vi "Secure-Release Region.vi"(6 "Numeric":dbl, 7 "Action":enum16{"Secure", "Release"}(ring), 8 "error in (no error)":errorcluster, 10 "Control In":T1={"I-O.lvclass"=refnum, "Gantry"=refnum, "Dispenser"="COM1"}, 11 "Workspace in":refnum<class "Component Tray.lvclass">) -> (0 "error out":errorcluster, 1 "Position":i32, 2 "Control Out":T1={"I-O.lvclass"=refnum, "Gantry"=refnum, "Dispenser"="COM1"}, 3 "Workspace out":refnum<class "Component Tray.lvclass">)   [LabVIEW 2021, in "Component Tray.lvclass"]
uses:
  Component Tray.lvclass
  C:/Users/HEP/Documents/GitHub/Gantry/UCSB-Gantry-HEP-main/Classes/Workspace/Fixture.lvclass
  Controller/Controllers.ctl
  Controller/I-O/I-O.lvclass
  C:/Program Files (x86)/Aerotech/A3200/LabVIEW/2010/Bin/Aerotech.A3200.dll
  Program Files (x86)/Aerotech/A3200/LabVIEW/2010/Bin/Aerotech.A3200.dll
  Fixture.lvclass/Fixture.ctl
  Read Gantry Region.vi
  Read Position.vi
  Fixture.lvclass
  Controller/Motion/Motion.lvclass
  Controller/Controller.lvclass
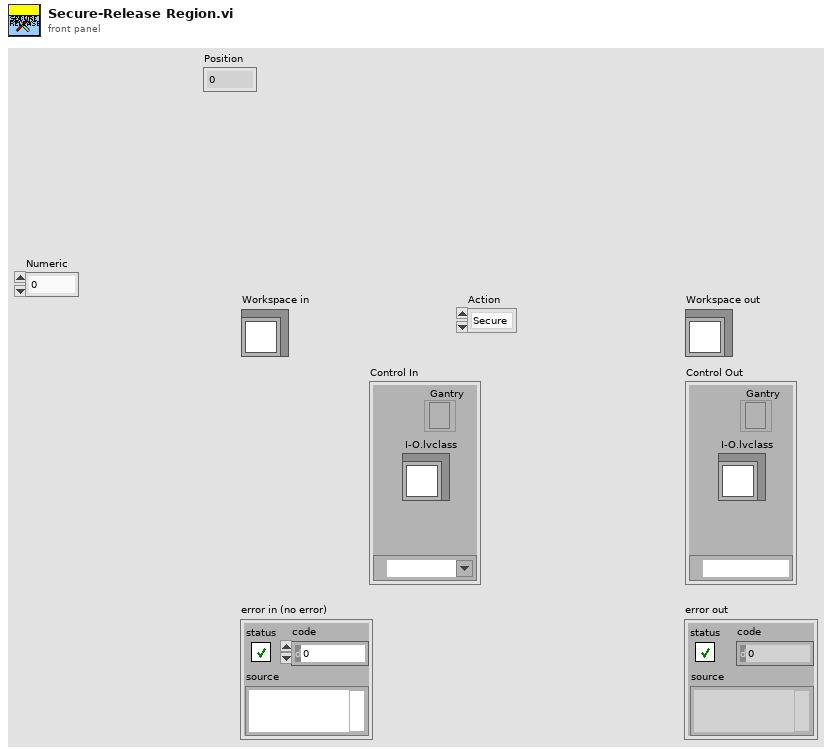
[diagram p1: front panel]
types:
  T1 = typedef "Controller.lvclass/Controllers.ctl" = cluster{"I-O.lvclass":refnum<class "I-O.lvclass">, "Gantry":refnum<k24>, "Dispenser":refnum<visa-resource-name>}
  T2 = typedef "I-O.lvclass/Pin Map.ctl" = cluster{"Region Valves":i32[], "Extra Valves":dbl[][][], "Tool Primary Valve":i32, "Tool Secondary Valve":i32, "Region Sensors":i32[], "Extra Sensors":dbl[][][], "Tool Primary Sensor":dbl, "Tool Secondary Sensor":dbl, "Compression Sensor":dbl, "5V":i32, "Dispenser Sensor":dbl}
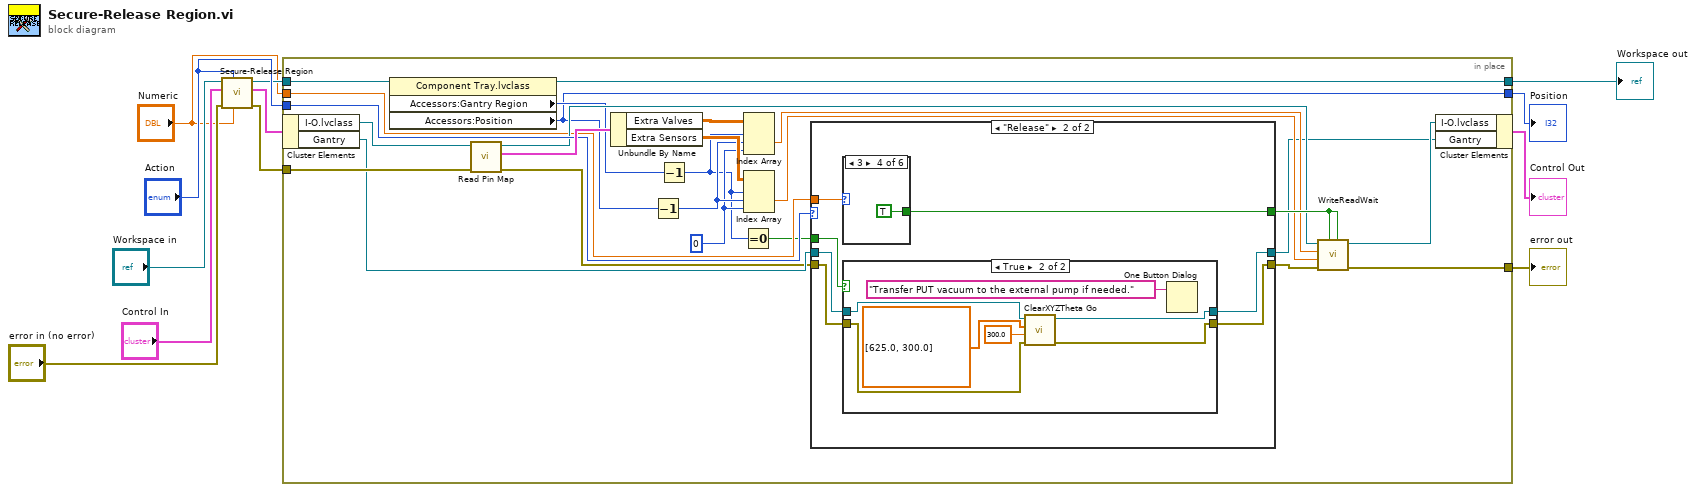
[diagram p0: block diagram]
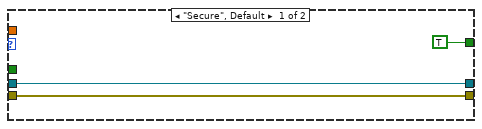
[diagram p2: hidden frame]
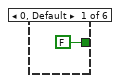
[diagram p4: hidden frame]
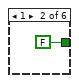
[diagram p5: hidden frame]
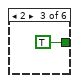
[diagram p6: hidden frame]
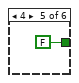
[diagram p7: hidden frame]
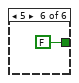
[diagram p8: hidden frame]
diagram:
  n1 = call-parent "Secure-Release Region.vi"("Test Run Number"="Numeric", "Action"="Action", "error in (no error)"="error in (no error)", "Control In"="Control In", "Fixture in"="Workspace in") -> ("error out"=w2:errorcluster, "Control Out"=w9:T1, "Fixture out"=w6:refnum<class "Component Tray.lvclass">)  [unwired: 3 in, 1 out]
  n2 = in-place {
    in-place-border: "Action" -> [w34]
    in-place-border: w6 -> [w31]
    in-place-border: [w26] -> w5
    in-place-border: [w22] -> w4
    in-place-border: "Numeric" -> [w21]
    in-place-border: w2 -> [w19]
    in-place-border: [w18] -> w1
    w23 = 0
    n3 = in-place-cluster #1(w9) -> ("I-O.lvclass"=w36:refnum<class "I-O.lvclass">, "Gantry"=w16:refnum<k24>)
    n4 = property class="Component Tray.lvclass"(reference=w31) -> (reference out=w26:refnum<class "Component Tray.lvclass">, "Accessors:Gantry Region"=w28:i32, "Accessors:Position"=w22:i32)  [unwired: 1 in, 1 out]
    n5 = call-dynamic "Read Pin Map.vi"("error in (no error)"=w19, "I-O in"=w36) -> ("error out"=w15:errorcluster, "Pin Map 2"=w37:T2, "I-O out"=w33:refnum<class "I-O.lvclass">)  [unwired: 7 in]
    n6 = Unbundle By Name(w37) -> ("Extra Valves"=w30:dbl[][][], "Extra Sensors"=w29:dbl[][][])
    n7 = Decrement(x=w22) -> (x-1=w27:i32)
    n8 = Decrement(x=w28) -> (x-1=w20:i32)
    n9 = Equal To 0?(x=w20) -> (x = 0?=w17:bool)
    n10 = Index Array(array=w30, index (dim 0)=w20, index (dim 1)=w27, index (dim 2)=w23) -> (element=w25:dbl)
    n11 = Index Array(array=w29, index (dim 0)=w20, index (dim 1)=w27, index (dim 2)=w23) -> (element=w24:dbl)
    n12 = case shown="\"Release\"" w34 {
      tunnel: [TRUE w46] -> w35
      tunnel: w21 -> [_ w47]
      tunnel: w17 -> [_ w45]
      tunnel: w16 -> [w39 w44]
      tunnel: w15 -> [w38 w43]
      tunnel: [w39 w42] -> w14
      tunnel: [w38 w41] -> w13
      frame "Secure", Default {
      }
      frame "Release" {
        n13 = case shown="3" w47 {
          tunnel: [FALSE FALSE TRUE TRUE FALSE FALSE] -> w46
          frame 0, Default {
          }
          frame 1 {
          }
          frame 2 {
          }
          frame 3 {
          }
          frame 4 {
          }
          frame 5 {
          }
        }
        n14 = case shown="True" w45 {
          tunnel: w44 -> [w49 w53]
          tunnel: [w49 w52] -> w42
          tunnel: w43 -> [w48 w51]
          tunnel: [w48 w50] -> w41
          frame False {
          }
          frame True {
            n15 = call "ClearXYZTheta Go.vi"("error in (no error)"=w51, "Speed"=300.0, "XYZTheta In"=dbl[] [625.0, 300.0], "Gantry In"=w53) -> ("error out"=w50:errorcluster, "Gantry Out"=w52:refnum<k24>)  [unwired: 5 in, 1 out]
            n16 = One Button Dialog(message="Transfer PUT vacuum to the external pump if needed.") -> ()  [unwired: 1 in, 1 out]
          }
        }
      }
    }
    n17 = call "WriteReadWait.vi"("Read Value"=w35, "Write Value"=w35, "error in (no error)"=w13, "Read"=w24, "Write"=w25, "I-O in"=w33) -> ("error out"=w18:errorcluster, "I-O out"=w32:refnum<class "I-O.lvclass">)  [unwired: 4 in]
    n18 = in-place-cluster #1("I-O.lvclass"=w32, "Gantry"=w14) -> (→"Control Out":T1)
  }
  "error out" <- w1
  "Workspace out" <- w5
  "Position" <- w4
